vi "Prober_InitialiseUI.vi"(8 "error in (no error)":errorcluster, 11 "AlessiRel6100 in":refnum<class "AlessiRel6100.lvclass">) -> (0 "error out":errorcluster, 2 "Probestation Configuration":variant, 3 "AlessiRel6100 out":refnum<class "AlessiRel6100.lvclass">)   [LabVIEW 2018, in "AlessiRel6100.lvclass"]
uses:
  AlessiRel6100.lvclass
  C:/Users/itk/Documents/itk-strip-sensor-qc/InstrControl/ProbeStationControl/ProbeStationControl.lvclass
  Alessi.vi
  QCtests/general_VIs/globals/QC_MeasurementSetup.vi
panel:
  in  "Touchdown method":enum16{"no feedback", "Arduino edgesense"}(ring)=enum."Arduino edgesense"
  in  "Overdrive [µm]":i32=30
  in  "Speed [µm/step]":i32=20
  in  "Search Band [µm]":i32=100
  in  "Edgesense params":T1={"touchdown height [µm]"=0, "search band [µm]"=100, "speed [µm/step]"=10, "overdrive [µm]"=30}
  out "Device ID":u32=2
  out "Ref No.":u32
  in  "Needles Clear":bool
  in  "Nucleus":bool
  in  "Stop Button":bool
  # "Starting Probe Station Control Interface"
  # "Arduino Edgesense"
  # "Before continuing, please confirm the following:"
  # "1. NUCLEUS is activiated"
  # "2. No device on chuck and needles are clear"
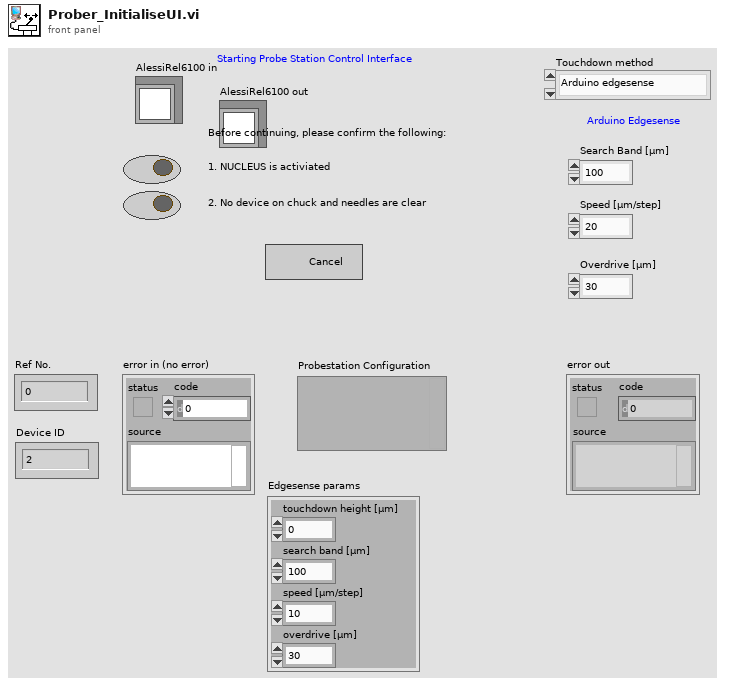
[diagram p1: front panel]
types:
  T1 = cluster{"touchdown height [µm]":i32, "search band [µm]":u32, "speed [µm/step]":u32, "overdrive [µm]":u32}
  T2 = cluster{"Device ID Probe Station":u32, "Ref No.":u32, "Touchdown method":enum16{"no feedback", "Arduino edgesense"}, "Arduino Edgesense params":cluster{"touchdown height [µm]":i32, "search band [µm]":u32, "speed [µm/step]":u32, "overdrive [µm]":u32}}
  T3 = cluster{"Bias Supply":refnum<class "SupplyControl.lvclass">, "SMU":refnum<class "SupplyControl.lvclass">, "LCR":refnum<class "LCRControl.lvclass">, "Probe Card Channels":i32, "Bias Voltage [V]":dbl, "First strip":i32, "Last strip":i32, "Base Voltage [V]":dbl, "Base Ramp Step [V]":dbl, "Base Ramp Interval [ms]":u32, "High Voltage [V]":dbl, "High Ramp Step [V]":dbl, "High Ramp Interval [ms]":u32, "Single Needle":bool, "Temperature Readout":enum16{"Read Arduino", "Enter manually"}, "Arduino":refnum<class "ArduinoControl.lvclass">, "Fraction of good strips [%]":dbl, "ProbeStation":refnum<class "ProbeStationControl.lvclass">, "AC frequency [Hz]":i32, "Switching":refnum<class "Switching.lvclass">, "Matrix used?":bool, "Matrix X Channels":cluster{"Bias Supply / SMU LO":i32, "Bias Supply / SMU HI":i32, "CV Box LO":i32, "CV Box HI":i32, "CV Box LO IN":i32, "CV Box HI IN":i32, "Volt meter LO":i32, "Volt meter HI":i32, "Mux1 C1":i32, "Mux1 C2":i32, "Mux2 C1":i32, "Mux2 C2":i32}, "Pinholes Y/N":bool, "Capacitance Y/N":bool, "Resistance Y/N":bool}
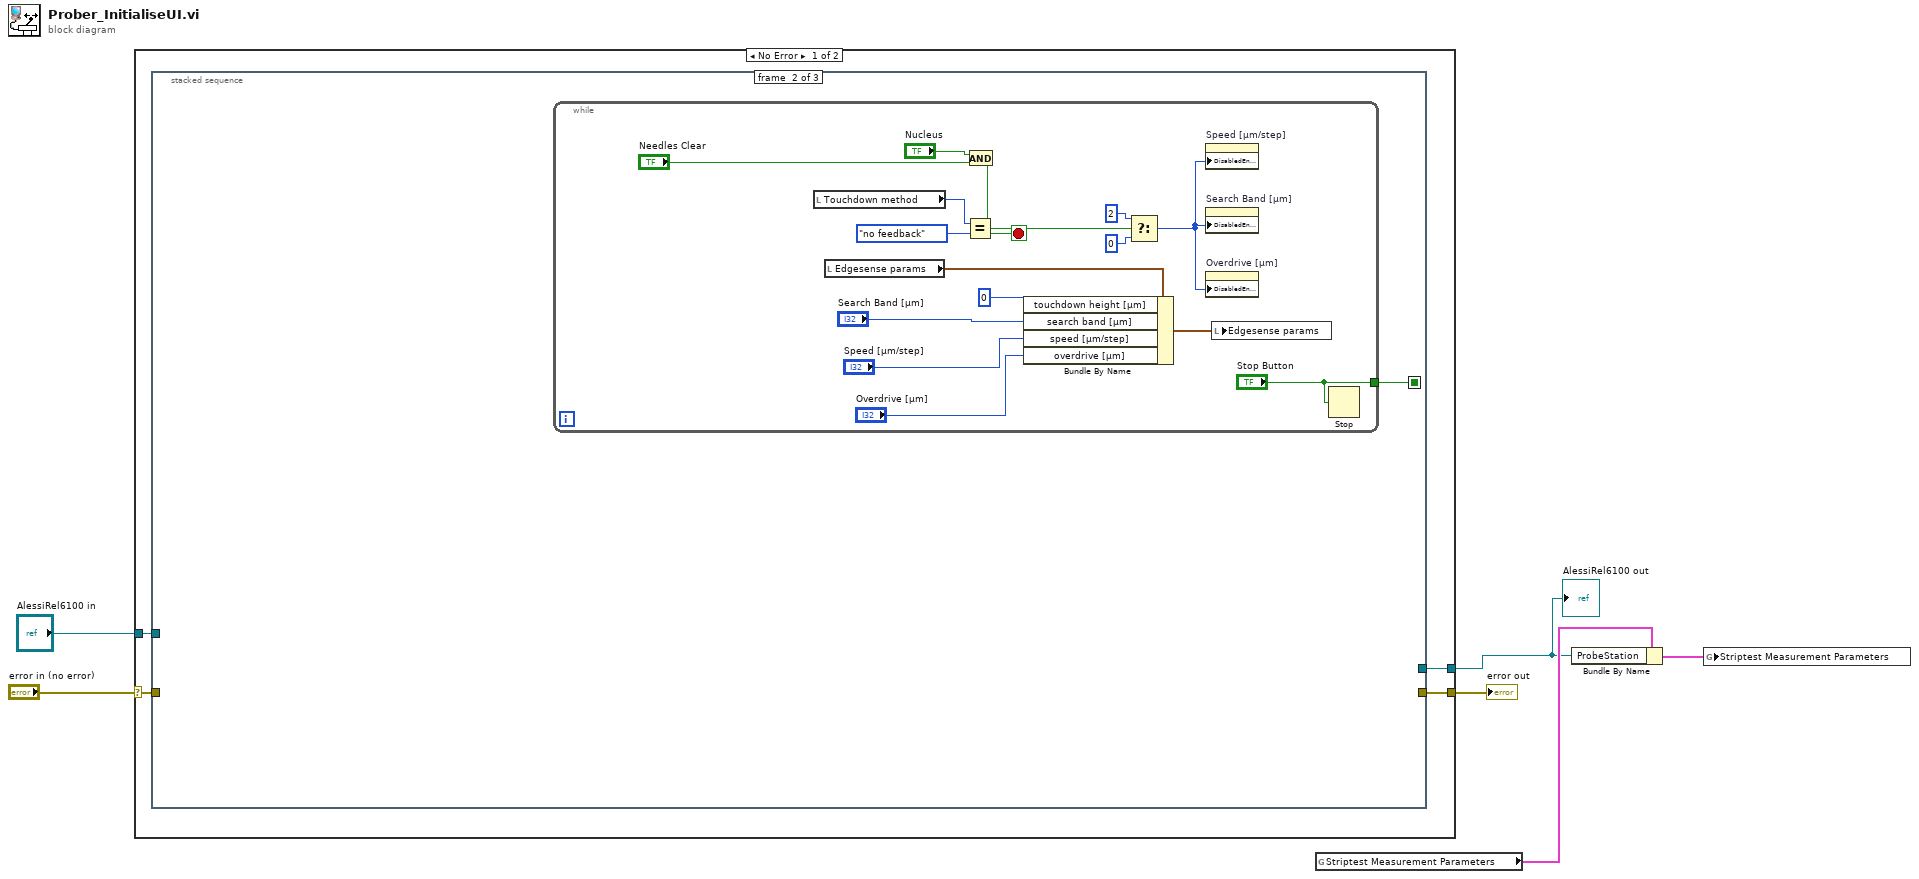
[diagram p0: block diagram]
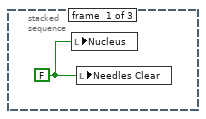
[diagram p2: hidden frame]
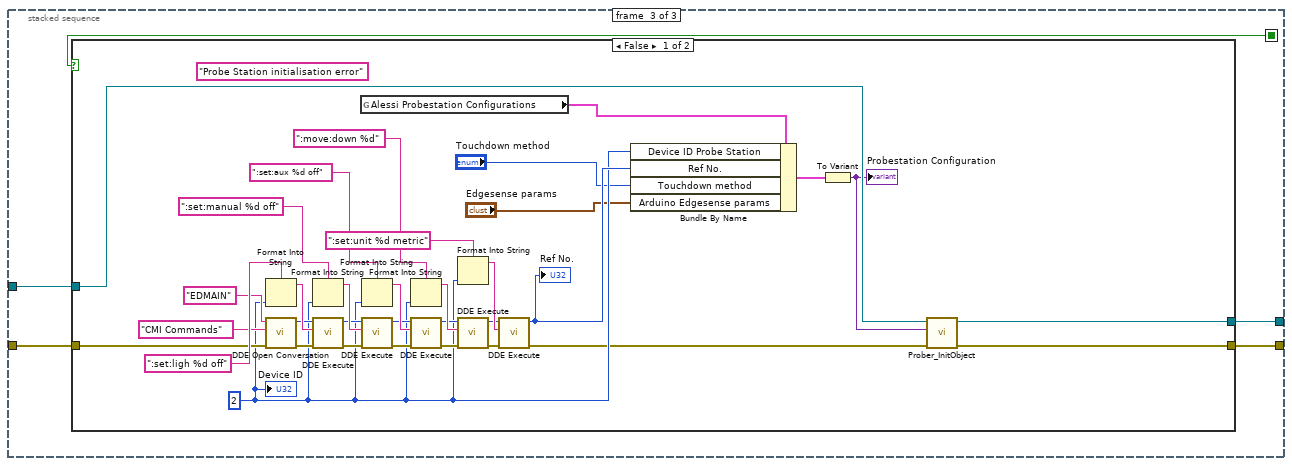
[diagram p3: hidden frame]
diagram:
  n1 = case shown="No Error" "error in (no error)" {
    selector: "error in (no error)" -> [w10 w71]
    tunnel: [w8 w71] -> w4
    tunnel: "AlessiRel6100 in" -> [w9 w70]
    tunnel: [w7 w70] -> w1
    frame No Error {
      n2 = stacked-sequence {
        seq-local: [_ w12 _] -> [_ _ w33]
        tunnel: w10 -> [_ _ w31]
        tunnel: w9 -> [_ _ w32]
        tunnel: [_ _ w30] -> w8
        tunnel: [_ _ w29] -> w7
        frame #0 {
          w11 = FALSE
          n3 = local write "Nucleus"(w11) -> ()
          n4 = local write "Needles Clear"(w11) -> ()
        }
        frame #1 {
          n5 = while {
            tunnel: ["Stop Button"] -> w12
            stop <- w28 stop-if-true
            n6 = local read "Touchdown method"() -> (w17:enum16{"no feedback", "Arduino edgesense"})
            n7 = local read "Edgesense params"() -> (w20:T1)
            n8 = Equal?(x=w17, y=enum16{"no feedback", "Arduino edgesense"}."no feedback" ("Touchdown method")) -> (x = y?=w16:bool)
            n9 = And(x="Nucleus", y="Needles Clear") -> (x .and. y?=w28:bool)
            n10 = Bundle By Name(cluster=w20, "touchdown height [µm]"=0, "search band [µm]"="Search Band [µm]", "speed [µm/step]"="Speed [µm/step]", "overdrive [µm]"="Overdrive [µm]") -> (w19:T1)
            n11 = Select(t=2, s=w16, f=0) -> (s? t:f=w13:i32)
            n12 = property on="Speed [µm/step]" class="DigNum (strict)"("DisabledEnum"=w13) -> ()  [unwired: 2 in, 2 out]
            n13 = property on="Search Band [µm]" class="DigNum (strict)"("DisabledEnum"=w13) -> ()  [unwired: 2 in, 2 out]
            n14 = property on="Overdrive [µm]" class="DigNum (strict)"("DisabledEnum"=w13) -> ()  [unwired: 2 in, 2 out]
            n15 = local write "Edgesense params"(w19) -> ()
            n16 = Stop(stop? (T)="Stop Button") -> ()
          }
        }
        frame #2 {
          n17 = case shown="False" w33 {
            tunnel: w32 -> [w43 w68]
            tunnel: w31 -> [w42 w69]
            tunnel: [w38 w69] -> w30
            tunnel: [w40 w68] -> w29
            frame False {
              w41 = u32 2
              (unwired) "Probe Station initialisation error" ("Error String IN")
              n18 = Format Into String(format string=":set:ligh %d off", w41) -> (resulting string=w63:string)  [unwired: 2 in, 1 out]
              n19 = call "DDE Open Conversation.vi"("error in (no error)"=w42, "topic"="CMI Commands", "service"="EDMAIN") -> ("error out"=w47:errorcluster, "conversation refnum"=w46:u32)  [unwired: 5 in]
              n20 = Format Into String(format string=":set:manual %d off" ("command"), w41) -> (resulting string=w60:string)  [unwired: 2 in, 1 out]
              n21 = call "DDE Execute.vi"("error in (no error)"=w47, "command"=w63, "conversation refnum in"=w46) -> ("error out"=w51:errorcluster, "conversation refnum out"=w48:u32)  [unwired: 5 in]
              n22 = global read "Alessi.vi" "Alessi Probestation Configurations"() -> (w35:T2)
              n23 = Format Into String(format string=":set:aux %d off" ("command"), w41) -> (resulting string=w61:string)  [unwired: 2 in, 1 out]
              n24 = call "DDE Execute.vi"("error in (no error)"=w51, "command"=w60, "conversation refnum in"=w48) -> ("error out"=w52:errorcluster, "conversation refnum out"=w49:u32)  [unwired: 5 in]
              n25 = Format Into String(format string=":move:down %d" ("command"), w41) -> (resulting string=w62:string)  [unwired: 2 in, 1 out]
              n26 = call "DDE Execute.vi"("error in (no error)"=w52, "command"=w61, "conversation refnum in"=w49) -> ("error out"=w53:errorcluster, "conversation refnum out"=w50:u32)  [unwired: 5 in]
              n27 = Format Into String(format string=":set:unit %d metric" ("command"), w41) -> (resulting string=w67:string)  [unwired: 2 in, 1 out]
              n28 = call "DDE Execute.vi"("error in (no error)"=w53, "command"=w62, "conversation refnum in"=w50) -> ("error out"=w64:errorcluster, "conversation refnum out"=w65:u32)  [unwired: 5 in]
              n29 = call "DDE Execute.vi"("error in (no error)"=w64, "command"=w67, "conversation refnum in"=w65) -> ("error out"=w39:errorcluster, "conversation refnum out"=w45:u32)  [unwired: 5 in]
              "Ref No." <- w45
              n30 = Bundle By Name(cluster=w35, "Device ID Probe Station"=w41, "Ref No."=w45, "Touchdown method"="Touchdown method", "Arduino Edgesense params"="Edgesense params") -> (w44:T2)
              n31 = To Variant(anything=w44) -> (Variant=w34:variant)
              "Probestation Configuration" <- w34
              n32 = call-dynamic "Prober_InitObject.vi"("error in (no error)"=w39, "Prober Configuration"=w34, "AlessiRel6100 in"=w43) -> ("error out"=w38:errorcluster, "AlessiRel6100 out"=w40:refnum<class "AlessiRel6100.lvclass">)  [unwired: 7 in]
              "Device ID" <- w41
            }
            frame True {
            }
          }
        }
      }
    }
    frame Error {
    }
  }
  "error out" <- w4
  "AlessiRel6100 out" <- w1
  n33 = global read "QC_MeasurementSetup.vi" "Striptest Measurement Parameters"() -> (w3:T3)
  n34 = Bundle By Name(cluster=w3, "ProbeStation"=w1) -> (w2:T3)
  n35 = global write "QC_MeasurementSetup.vi" "Striptest Measurement Parameters"(w2) -> ()
